vi "Dequeue Message (enum).vi"(8 "error in (no error)":errorcluster, 9 "timeout in ms (-1)":i32, 11 "Message Queue":refnum<queue>) -> (0 "error out":errorcluster, 1 "Message Data":variant, 2 "Enum":T1, 3 "dup Message Queue":refnum<queue>)   [LabVIEW 2018, in "Message Queue.lvlib"]
doc: "This VI pulls messages off the Message Queue. It has special error handling to account for an error occurring on the last iteration of the Message Handling Loop.\n\nNo Error - normal Dequeue Element operation.\nError - check if it is an error code we wish to ignore. If so, clear the error and perform a normal Dequeue Element. If not, output the error, and put a 'Stop' message on the Message Queue."
uses:
  Message Queue.lvlib
  Message Cluster (enum).ctl
  Message (enum).ctl
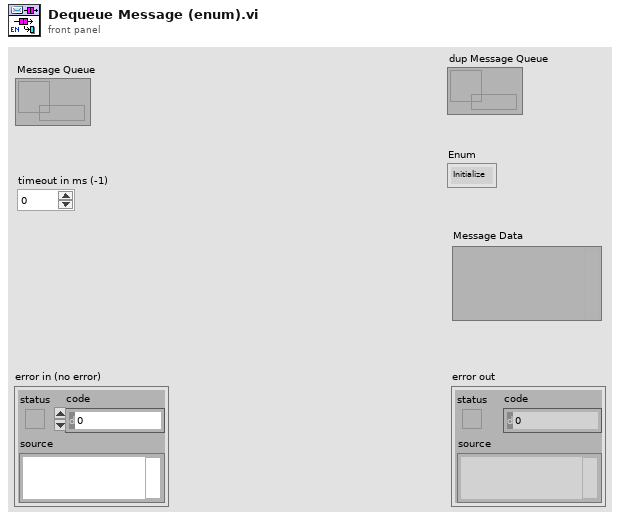
[diagram p1: front panel]
types:
  T1 = typedef "Message Queue.lvlib/Message (enum).ctl" = enum16{"Initialize", "Idle", "Running", "Stop", "Pause", "Resume", "Load Sequence File", "Load Sequence from UI", "Save Sequence File"}
  T2 = typedef "Message Queue.lvlib/Message Cluster (enum).ctl" = cluster{"Message":T1, "Message Data":variant}
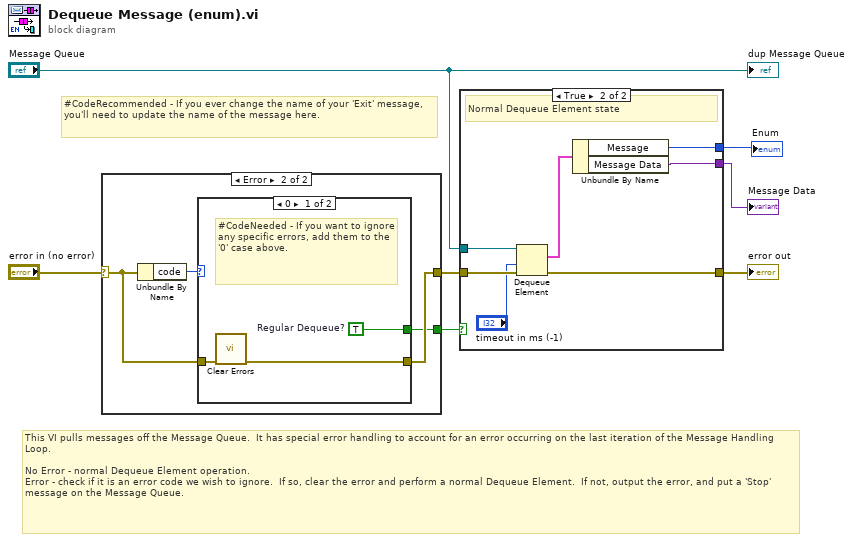
[diagram p0: block diagram]
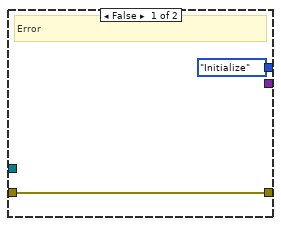
[diagram p2: hidden frame]
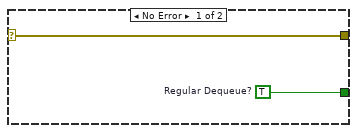
[diagram p3: hidden frame]
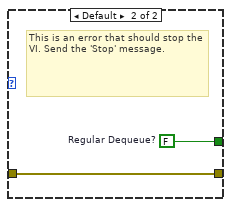
[diagram p4: hidden frame]
diagram:
  # "#CodeRecommended - If you ever change the name of your 'Exit' message, you'll need to update the name of the message here."
  # "This VI pulls messages off the Message Queue.  It has special error handling to account for an error occurring on the last iteration of the Message Handling Loop.\n\nNo Error - normal Dequeue Element operation.\nError - check if it is an error code we wish to ignore.  If so, clear the error and perform a normal Dequeue Element.  If not, output the error, and put a 'Stop' message on the Message Queue."
  n1 = case shown="Error" "error in (no error)" {
    selector: "error in (no error)" -> [w9 w12]
    tunnel: [w9 w11] -> w5
    tunnel: [w8 w10] -> w4
    frame No Error {
      w8 = TRUE  # Regular Dequeue?
    }
    frame Error {
      n2 = Unbundle By Name(w12) -> ("code"=w13:i32)
      n3 = case shown="0" w13 {
        tunnel: [w16 w18] -> w11
        tunnel: w12 -> [w15 w18]
        tunnel: [w14 w17] -> w10
        frame 0 {
          w14 = TRUE  # Regular Dequeue?
          # "#CodeNeeded - If you want to ignore any specific errors, add them to the '0' case above."
          n4 = call <vilib>:"Clear Errors.vi"("error in (no error)"=w15) -> ("error out"=w16:errorcluster)  [unwired: 5 in, 1 out]
        }
        frame Default {
          w17 = FALSE  # Regular Dequeue?
          # "This is an error that should stop the VI. Send the 'Stop' message."
        }
      }
    }
  }
  n5 = case shown="True" w4 {
    tunnel: [w20 w27] -> w6
    tunnel: w5 -> [w20 w26]
    tunnel: "Message Queue" -> [_ w25]
    tunnel: [_ w23] -> w2
    tunnel: [Message_(enum)."Initialize" ("Message") w22] -> w1
    frame False {
      # "Error"
    }
    frame True {
      # "Normal Dequeue Element state"
      n6 = Dequeue Element(queue=w25, timeout in ms (-1)="timeout in ms (-1)", error in (no error)=w26) -> (element=w24:T2, error out=w27:errorcluster)  [unwired: 2 out]
      n7 = Unbundle By Name(w24) -> ("Message"=w22:T1, "Message Data"=w23:variant)
    }
  }
  "error out" <- w6
  "Message Data" <- w2
  "Enum" <- w1
  "dup Message Queue" <- "Message Queue"
